vi "PAC_load_VI.vi"(8 "error in (no error)":errorcluster, 11 "Barcode":string) -> (0 "error out":errorcluster)   [LabVIEW 2024, in "Test_2.lvlib"]
uses:
  Test_2.lvlib
  Launcher/Launcher_DTU.lvlib
panel:
  out "6th letter":string
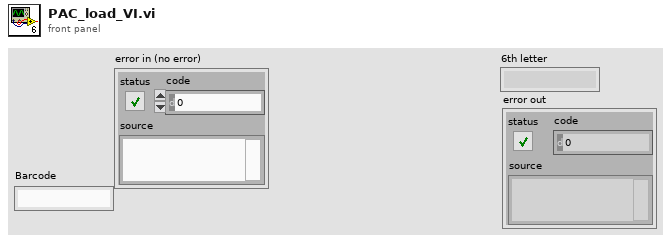
[diagram p1: front panel]
types:
  T1 = enum16{"Read", "Write", "All_sections", "All_values", "Remove key&section"}
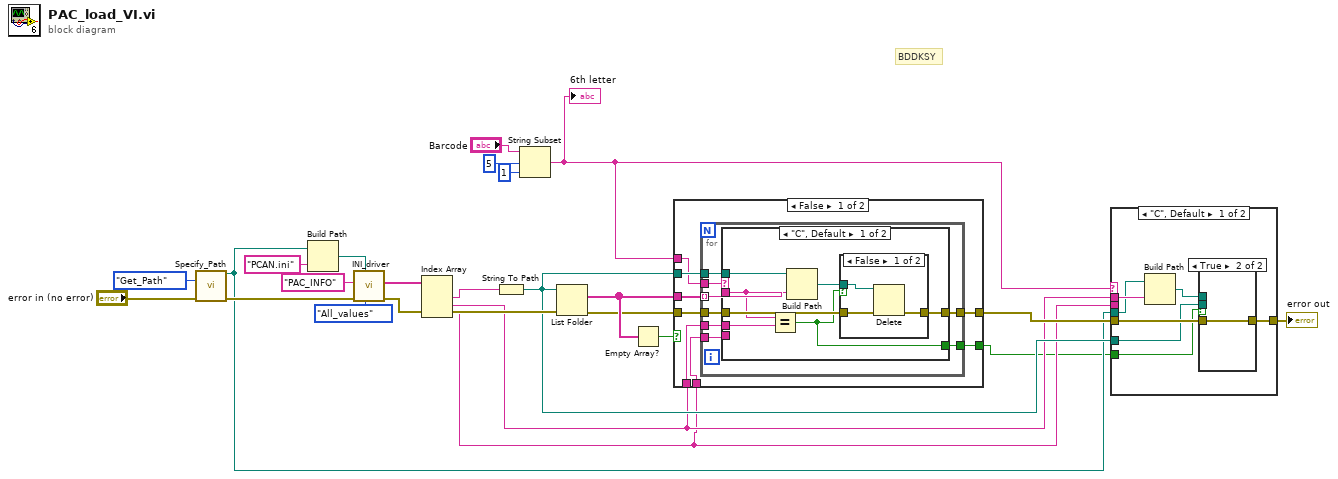
[diagram p0: block diagram]
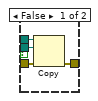
[diagram p2: hidden frame]
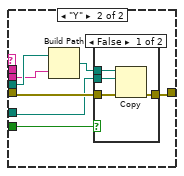
[diagram p3: hidden frame]
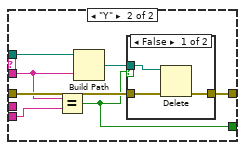
[diagram p6: hidden frame]
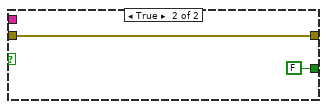
[diagram p8: hidden frame]
diagram:
  # "BDDKSY"
  n1 = call "Specify_Path.vi"("Path_Enum"=enum16{"Find_Path", "Get_Path"}."Get_Path", "error in (no error)"="error in (no error)") -> ("Configurations"=w7:path, "error out"=w20:errorcluster)  [unwired: 6 in, 6 out]
  n2 = Build Path(base path=w7, name or relative path="PCAN.ini") -> (appended path=w18:path)
  n3 = call "INI_driver.vi"("Enum"=T1."All_values", "instrument file path"=w18, "error in (no error)"=w20, "Section"="PAC_INFO") -> ("error out"=w11:errorcluster, "Values out"=w15:string[])  [unwired: 4 in, 2 out]
  n4 = Index Array(array=w15) -> (element #1=w14:string, element #2=w3:string, element #3=w2:string)  [unwired: 3 in]
  n5 = String To Path(string=w14) -> (path=w9:path)
  n6 = String Subset(string="Barcode", offset (0)=5, length (rest)=1 ("length (rest)")) -> (substring=w4:string)
  "6th letter" <- w4
  n7 = List Folder(path=w9, error in=w11) -> (filenames=w13:string[], error out=w10:errorcluster)  [unwired: 2 in, 2 out]
  n8 = Empty Array?(array=w13) -> (empty?=w12:bool)
  n9 = case shown="False" w12 {
    tunnel: w9 -> [w32 _]
    tunnel: w13 -> [w31 _]
    tunnel: w10 -> [w30 w64]
    tunnel: [w29 w64] -> w8
    tunnel: w4 -> [w28 _]
    tunnel: w3 -> [w27 _]
    tunnel: w2 -> [w26 _]
    tunnel: [w25 FALSE] -> w1
    frame False {
      n10 = for {
        tunnel: w31 -> [w39] mode=indexing
        tunnel: w32 -> [w40]
        tunnel: w30 -> [w38]
        tunnel: [w37] -> w29
        tunnel: w28 -> [w36]
        tunnel: w27 -> [w35]
        tunnel: w26 -> [w34]
        tunnel: [w33] -> w25
        n11 = case shown="\"C\", Default" w36 {
          tunnel: w40 -> [w47 w58]
          tunnel: w39 -> [w43 w54]
          tunnel: w38 -> [w45 w56]
          tunnel: [w44 w55] -> w37
          tunnel: w35 -> [w42 _]
          tunnel: w34 -> [_ w53]
          tunnel: [w41 w52] -> w33
          frame "C", Default {
            n12 = Equal?(x=w43, y=w42) -> (x = y?=w41:bool)
            n13 = Build Path(base path=w47, name or relative path=w43) -> (appended path=w46:path)
            n14 = case shown="False" w41 {
              tunnel: w46 -> [w50 _]
              tunnel: w45 -> [w49 w51]
              tunnel: [w48 w51] -> w44
              frame False {
                n15 = Delete(path (use dialog)=w50, error in=w49) -> (error out=w48:errorcluster)  [unwired: 3 in, 2 out]
              }
              frame True {
              }
            }
          }
          frame "Y" {
            n16 = Equal?(x=w54, y=w53) -> (x = y?=w52:bool)
            n17 = Build Path(base path=w58, name or relative path=w54) -> (appended path=w57:path)
            n18 = case shown="False" w52 {
              tunnel: w57 -> [w61 _]
              tunnel: w56 -> [w60 w62]
              tunnel: [w59 w62] -> w55
              frame False {
                n19 = Delete(path (use dialog)=w61, error in=w60) -> (error out=w59:errorcluster)  [unwired: 3 in, 2 out]
              }
              frame True {
              }
            }
          }
        }
      }
    }
    frame True {
    }
  }
  n20 = case shown="\"C\", Default" w4 {
    tunnel: w9 -> [w67 w81]
    tunnel: w8 -> [w71 w82]
    tunnel: w3 -> [w70 _]
    tunnel: w2 -> [_ w79]
    tunnel: w7 -> [w69 w80]
    tunnel: [w66 w78] -> w6
    tunnel: w1 -> [w65 w77]
    frame "C", Default {
      n21 = Build Path(base path=w69, name or relative path=w70) -> (appended path=w68:path)
      n22 = case shown="True" w65 {
        tunnel: w71 -> [w75 w76]
        tunnel: w68 -> [w74 _]
        tunnel: w67 -> [w73 _]
        tunnel: [w72 w76] -> w66
        frame False {
          n23 = Copy(8:w75, 10:w73, 11:w74) -> (0:w72:errorcluster)  [unwired: 2 in, 2 out]
        }
        frame True {
        }
      }
    }
    frame "Y" {
      n24 = Build Path(base path=w80, name or relative path=w79) -> (appended path=w83:path)
      n25 = case shown="False" w77 {
        tunnel: w83 -> [w87 _]
        tunnel: w82 -> [w86 w88]
        tunnel: w81 -> [w85 _]
        tunnel: [w84 w88] -> w78
        frame False {
          n26 = Copy(8:w86, 10:w85, 11:w87) -> (0:w84:errorcluster)  [unwired: 2 in, 2 out]
        }
        frame True {
        }
      }
    }
  }
  "error out" <- w6
